vi "uEye_Basics.vi"() -> ()   [LabVIEW 2016]
uses:
  System.Windows.Forms
  C:/Program Files/National Instruments/LabVIEW 2016/instr.lib/IDS/ueye.NET/uEyeDotNet.dll
  Program Files/National Instruments/LabVIEW 2016/instr.lib/IDS/ueye.NET/uEyeDotNet.dll
panel:
  in  "mode":i32(ring) items=["BGRA8Packed"=0, "BGR8Packed"=1, "BGR565Packed"=2, "BGR5Packed"=3, "Mono8"=6, "SensorRaw8"=11, "UYVYPacked"=12, "UYVYMonoPacked"=13, "UYVYBayerPacked"=14, "CBYCRYPacked"=23, "BGRY8Packed"=24, "BGR10Packed"=25, "Mono12"=26, "SensorRaw12"=27, "Mono16"=28, "SensorRaw16"=29, "BGR12Unpacked"=30, "BGRA12Unpacked"=31, "Jpeg"=32, "SensorRaw10"=33, "Mono10"=34, "BGR10Unpacked"=35, "RGBA8Packed"=128, "RGB8Packed"=129, "RGBY8Packed"=152, "RGB10Packed"=153, "RGB12Unpacked"=158, "RGBA12Unpacked"=159, "RGB10Unpacked"=163, "RGB8Planar"=8321, "PreferPackedSourceFormat"=16384]
  in  "PictureBox":refnum<k24>(container)
  in  "Camera ID":i32 min=0 max=255
  in  "Number of images \nto capture":i32=25 min=1
  out "Error Out":errorcluster
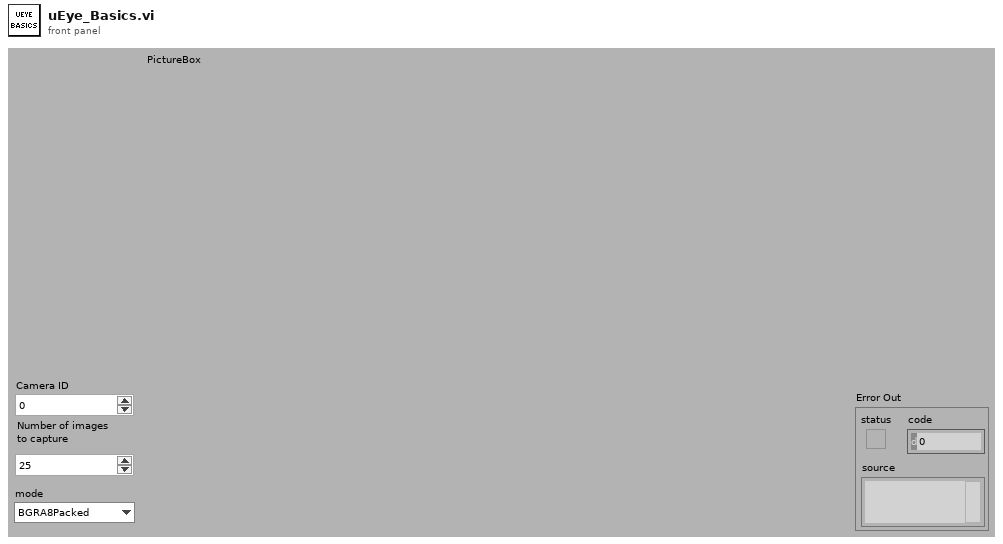
[diagram p1: front panel]
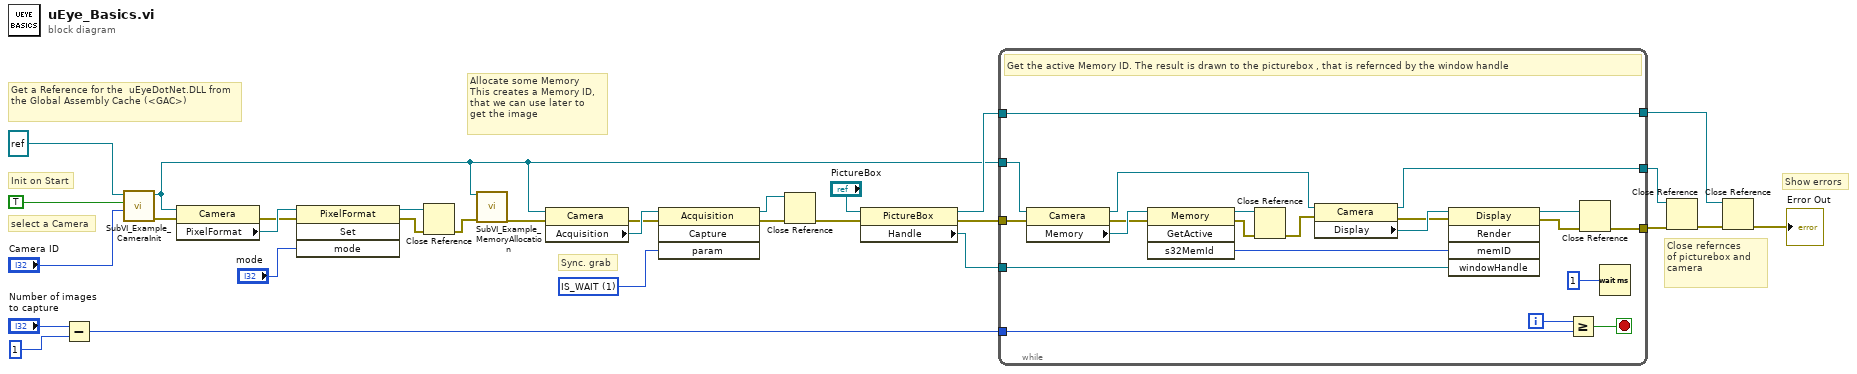
[diagram p0: block diagram]
diagram:
  w26 = 1 items=["IS_DONT_WAIT", "IS_WAIT"] ("Wait")
  # "Close refernces\nof picturebox and camera"
  # "Show errors"
  # "Allocate some Memory\nThis creates a Memory ID,\nthat we can use later to\nget the image"
  # "Sync. grab"
  # "select a Camera"
  # "Init on Start"
  # "Get a Reference for the  uEyeDotNet.DLL from the Global Assembly Cache (<GAC>)"
  n1 = Subtract(x="Number of images \nto capture", y=1) -> (x-y=w1:i32)
  n2 = call "SubVI_Example_CameraInit.vi"("Camera ID"="Camera ID", "Init Camera Flag"=TRUE ("Init Camera"), ".NET (Reference)"=refnum<k24> refnum (".NET (Referenz)")) -> ("Error Out"=w22:errorcluster, ".NET (Reference)"=w4:refnum<k24>)  [unwired: 7 in]
  n3 = property class="Camera"(reference=w4, error in=w22) -> (error out=w23:errorcluster, "PixelFormat"=w24:refnum<k24>)  [unwired: 1 out]
  n4 = invoke class="PixelFormat" method="Set"(reference=w24, error in=w23, "mode"="mode") -> (reference out=w15:refnum<k24>, error out=w14:errorcluster)  [unwired: 1 in, 2 out]
  n5 = Close Reference(reference=w15, error in (no error)=w14) -> (error out=w13:errorcluster)
  n6 = call "SubVI_Example_MemoryAllocation.vi"(".NET (Reference)"=w4, "Error In"=w13) -> ("Error Out"=w27:errorcluster)  [unwired: 13 in, 4 out]
  n7 = property class="Camera"(reference=w4, error in=w27) -> (error out=w28:errorcluster, "Acquisition"=w29:refnum<k24>)  [unwired: 1 out]
  n8 = invoke class="Acquisition" method="Capture"(reference=w29, error in=w28, "param"=w26) -> (reference out=w10:refnum<k24>, error out=w12:errorcluster)  [unwired: 1 in, 2 out]
  n9 = Close Reference(reference=w10, error in (no error)=w12) -> (error out=w11:errorcluster)
  n10 = property class="PictureBox"(reference="PictureBox", error in=w11) -> (reference out=w9:refnum<k24>, error out=w17:errorcluster, "Handle"=w16:refnum<k24>)
  n11 = while {
    tunnel: w17 -> [w48]
    tunnel: w4 -> [w35]
    tunnel: [w39] -> w20
    tunnel: [w38] -> w19
    tunnel: w16 -> [w37]
    tunnel: [w32] -> w6
    tunnel: w9 -> [w32]
    tunnel: w1 -> [w31]
    i -> [w47]
    stop <- w51 stop-if-true
    # "Get the active Memory ID. The result is drawn to the picturebox , that is refernced by the window handle"
    n12 = property class="Camera"(reference=w35, error in=w48) -> (reference out=w34:refnum<k24>, error out=w49:errorcluster, "Memory"=w50:refnum<k24>)
    n13 = invoke class="Memory" method="GetActive"(reference=w50, error in=w49) -> (reference out=w45:refnum<k24>, error out=w44:errorcluster, "s32MemId"=w36:i32)  [unwired: 2 in, 1 out]
    n14 = Close Reference(reference=w45, error in (no error)=w44) -> (error out=w43:errorcluster)
    n15 = property class="Camera"(reference=w34, error in=w43) -> (reference out=w38:refnum<k24>, error out=w42:errorcluster, "Display"=w46:refnum<k24>)
    n16 = invoke class="Display" method="Render"(reference=w46, error in=w42, "memID"=w36, "windowHandle"=w37) -> (reference out=w41:refnum<k24>, error out=w40:errorcluster)  [unwired: 1 in, 3 out]
    n17 = Greater Or Equal?(x=w47, y=w31) -> (x >= y?=w51:bool)
    n18 = Close Reference(reference=w41, error in (no error)=w40) -> (error out=w39:errorcluster)
    n19 = Wait (ms)(milliseconds to wait=u32 1) -> ()  [unwired: 1 out]
  }
  n20 = Close Reference(reference=w19, error in (no error)=w20) -> (error out=w8:errorcluster)
  n21 = Close Reference(reference=w6, error in (no error)=w8) -> (error out=→"Error Out":errorcluster)
